vi "test empty msg.vi"(8 "error in (no error)":errorcluster) -> (0 "error out":errorcluster, 3 "body":string)   [LabVIEW 2020, in "MCP Server tests.lvlib"]
uses:
  MCP Server tests.lvlib
  <vilib>/JDP Science/JSONtext/Next JSON Value.vi
  <vilib>/JDP Science/JSONtext/String Subset.vi
  <vilib>/JDP Science/JSONtext/Parsing/Advance past next JSON Value (inlined COPY).vi
  <vilib>/JDP Science/JSONtext/Parsing/Advance past whitespace.vi
  <vilib>/JDP Science/JSONtext/Parsing/Advance past String.vi
  <vilib>/JDP Science/JSONtext/Parsing/Advance past Number.vi
  <vilib>/JDP Science/JSONtext/Parsing/Advance past Line Ending.vi
  <vilib>/JDP Science/JSONtext/Parsing/Parse Full Path or Item Name.vi
  <vilib>/JDP Science/JSONtext/Parsing/Advance past Array.vi
  <vilib>/JDP Science/JSONtext/Parsing/Advance past Object.vi
  <vilib>/JDP Science/JSONtext/support/Error Cluster From Code.vi
  <vilib>/JDP Science/JSONtext/Offset/Find Item Locations by Path.vi
  <vilib>/addons/_JKI Toolkits/Caraya/classes/Test/Test.lvclass
  <vilib>/addons/_JKI Toolkits/Caraya/classes/Assert/Assert.lvclass
  <vilib>/JDP Science/JSONtext/JSONtext.lvlib
panel:
  out "headers":string
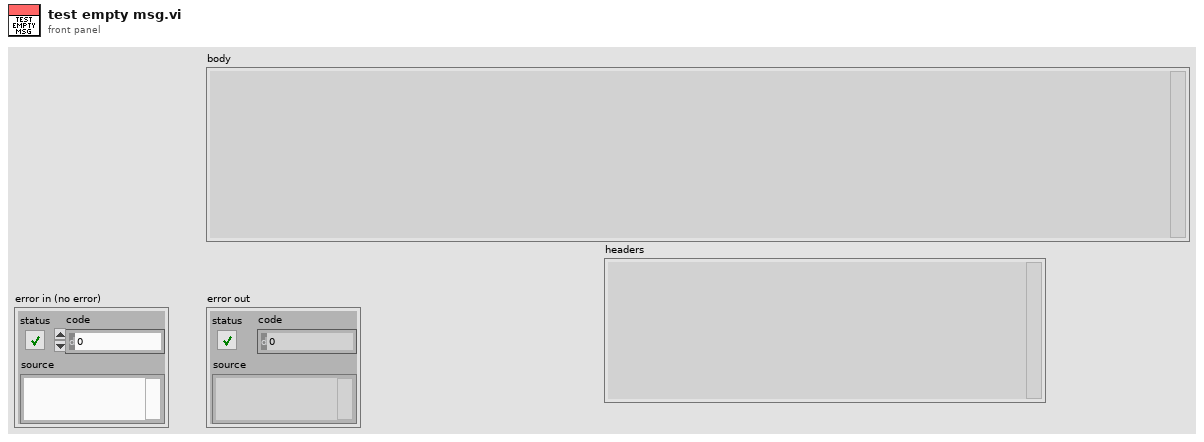
[diagram p1: front panel]
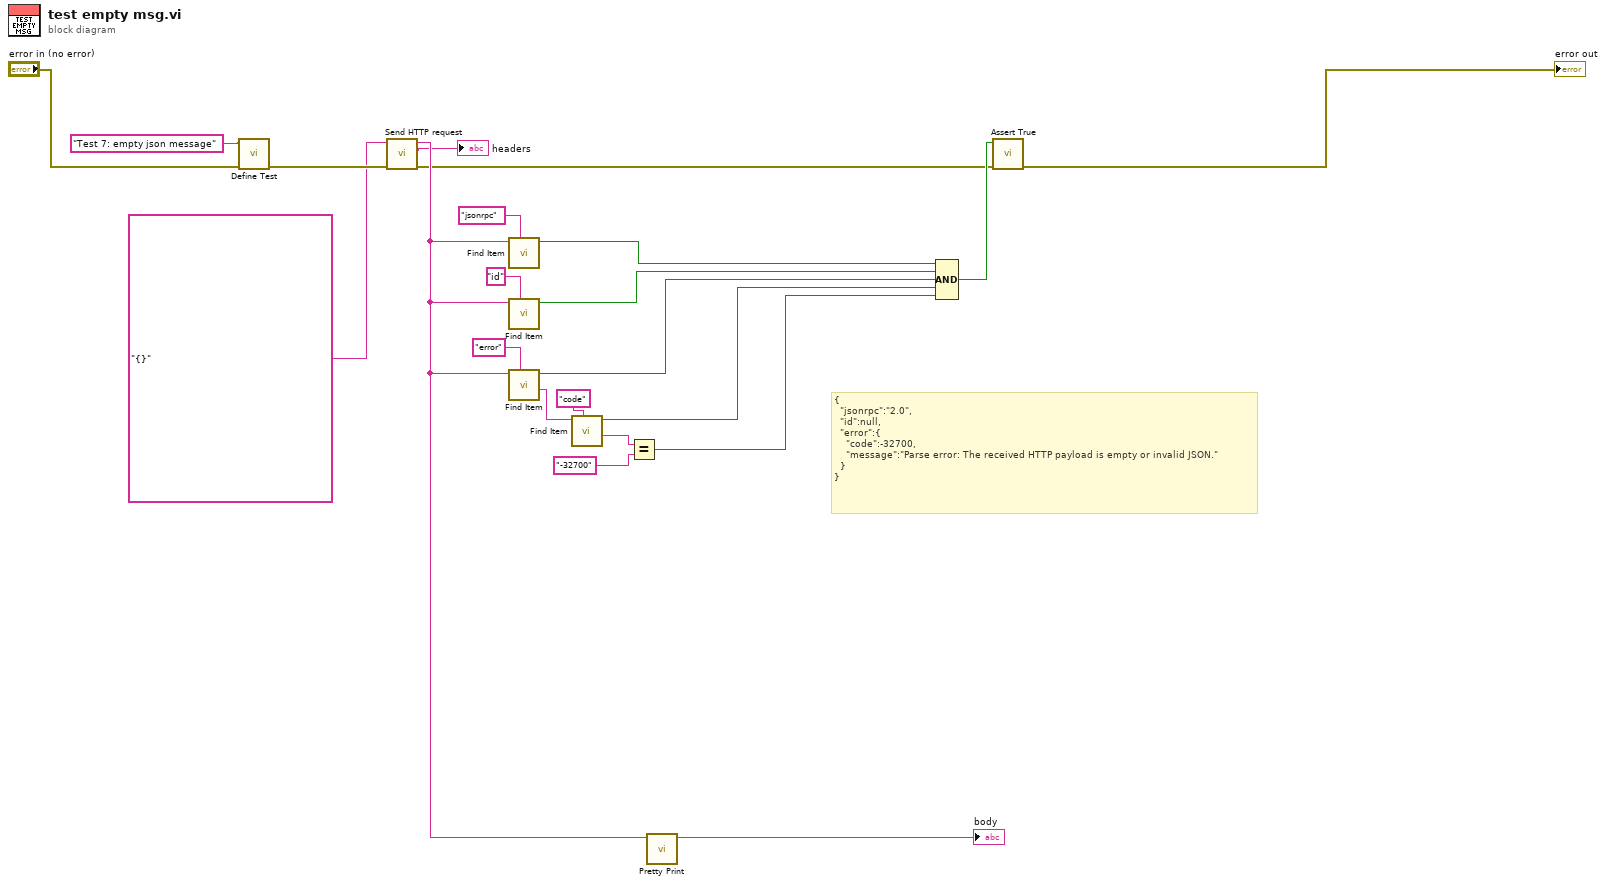
[diagram p0: block diagram]
diagram:
  # "{\n  \"jsonrpc\":\"2.0\",\n  \"id\":null,\n  \"error\":{\n    \"code\":-32700,\n    \"message\":\"Parse error: The received HTTP payload is empty or invalid JSON.\"\n  }\n}"
  n1 = call <vilib>:"Define Test.vi"("error in (no error)"="error in (no error)", "Label (VI Title)"="Test 7: empty json message") -> ("error out"=w12:errorcluster)  [unwired: 8 in, 1 out]
  n2 = call "Send HTTP request.vi"("error in (no error)"=w12, "request"="{}" ("buffer")) -> ("error out"=w13:errorcluster, "headers"=→"headers":string, "response"=w21:string)  [unwired: 7 in]
  n3 = call <vilib>:"Find Item.vi"("$Path or Item Name"="jsonrpc", "JSON"=w21) -> ("Found"=w16:bool)  [unwired: 6 in, 3 out]
  n4 = call <vilib>:"Find Item.vi"("$Path or Item Name"="id", "JSON"=w21) -> ("Found"=w17:bool)  [unwired: 6 in, 3 out]
  n5 = call <vilib>:"Find Item.vi"("$Path or Item Name"="error", "JSON"=w21) -> ("<JSON>"=w6:string, "Found"=w20:bool)  [unwired: 6 in, 2 out]
  n6 = call <vilib>:"Find Item.vi"("$Path or Item Name"="code", "JSON"=w6) -> ("<JSON>"=w4:string, "Found"=w2:bool)  [unwired: 6 in, 2 out]
  n7 = Equal?(x=w4, y="-32700") -> (x = y?=w1:bool)
  n8 = call <vilib>:"Pretty Print.vi"("JSON"=w21) -> ("<JSON>"=→"body":string)  [unwired: 8 in, 2 out]
  n9 = Compound Arithmetic op=AND(w16, w17, w20, w2, w1) -> (w18:bool)
  n10 = call <vilib>:"Assert True.vi"("error in (no error)"=w13, "True?"=w18) -> ("error out"=→"error out":errorcluster)  [unwired: 8 in, 1 out]
